vi "Read Msg Input.vi"(11 "Msg in":refnum<class "Msg.lvclass">) -> (2 "Msg Input":refnum<class "Msg Input.lvclass">)   [LabVIEW 2020, in "jettl.lvlib" / "Msg.lvclass"]
uses:
  Msg.lvclass
  Msg Input/Msg Input.lvclass
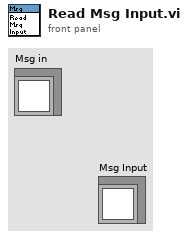
[diagram p1: front panel]
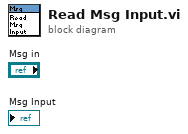
[diagram p0: block diagram]
diagram:
